vi "bit_to_rgb.vi"(11 "Slide":i32) -> (3 "Color":u32)   [LabVIEW 2017]
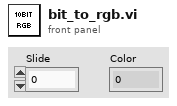
[diagram p1: front panel]
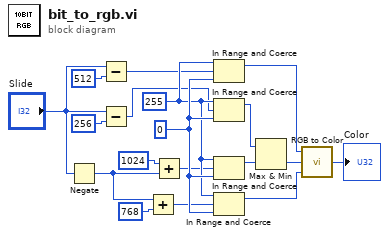
[diagram p0: block diagram]
diagram:
  w17 = 255
  w18 = 0
  n1 = Negate(x="Slide") -> (-x=w13:i32)
  n2 = Subtract(x="Slide", y=512) -> (x-y=w2:i32)
  n3 = Subtract(x="Slide", y=256) -> (x-y=w6:i32)
  n4 = Add(x=w13, y=768) -> (x+y=w14:i32)
  n5 = Add(x=1024, y=w13) -> (x+y=w7:i32)
  n6 = In Range and Coerce(upper limit=w17, x=w2, lower limit=w18) -> (coerced(x)=w9:i32)  [unwired: 1 out]
  n7 = In Range and Coerce(upper limit=w17, x=w6, lower limit=w18) -> (coerced(x)=w3:i32)  [unwired: 1 out]
  n8 = In Range and Coerce(upper limit=w17, x=w7, lower limit=w18) -> (coerced(x)=w5:i32)  [unwired: 1 out]
  n9 = In Range and Coerce(upper limit=w17, x=w14, lower limit=w18) -> (coerced(x)=w15:i32)  [unwired: 1 out]
  n10 = Max & Min(x=w3, y=w5) -> (min(x,y)=w10:i32)  [unwired: 1 out]
  n11 = call <vilib>:"RGB to Color.vi"("B"=w15, "G"=w10, "R"=w9) -> ("Color"=→"Color":u32)
